vi "SingleServiceRegistered_InvalidResolveRequests_Error.vi"(11 "error in":errorcluster) -> (6 "pass":bool, 8 "result":string, 15 "error out":errorcluster)   [LabVIEW 2020]
uses:
  Runtime/MeasurementLink Discovery Client/RPC Messages/ni_measurementlink_discovery_v1_RegisterServiceRequest.ctl
  Runtime/MeasurementLink Discovery Client/RPC Messages/ni_measurementlink_discovery_v1_ServiceDescriptor.ctl
  Runtime/MeasurementLink Discovery Client/RPC Messages/ni_measurementlink_discovery_v1_ServiceDescriptor_AnnotationsEntry.ctl
  Runtime/MeasurementLink Discovery Client/RPC Messages/ni_measurementlink_discovery_v1_ServiceLocation.ctl
  Runtime/MeasurementLink Discovery Client/RPC Messages/ni_measurementlink_discovery_v1_ResolveServiceRequest.ctl
  Runtime/MeasurementLink Discovery Client/MeasurementLink Discovery Client.lvlib
  Runtime/MeasurementLink Discovery V1/MeasurementLink Discovery V1.lvlib
panel:
  # "Test assumes discovery service has already been started."
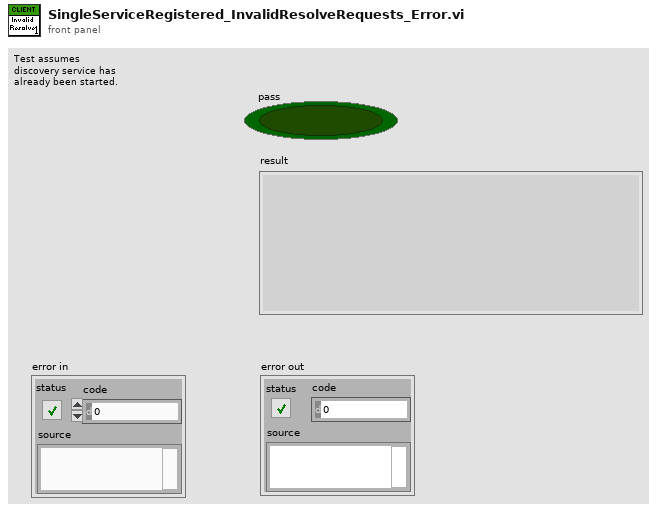
[diagram p1: front panel]
types:
  T1 = typedef "MeasurementLink Discovery Client.lvlib/ni_measurementlink_discovery_v1_ResolveServiceRequest.ctl" = cluster{"provided_interface":string, "service_class":string}
  T2 = typedef "MeasurementLink Discovery Client.lvlib/ni_measurementlink_discovery_v1_RegisterServiceRequest.ctl" = cluster{"service_description":T3, "location":T5}
  T3 = typedef "MeasurementLink Discovery Client.lvlib/ni_measurementlink_discovery_v1_ServiceDescriptor.ctl" = cluster{"display_name":string, "description_url":string, "provided_interfaces":string[], "service_class":string, "annotations":T4[]}
  T4 = typedef "MeasurementLink Discovery Client.lvlib/ni_measurementlink_discovery_v1_ServiceDescriptor_AnnotationsEntry.ctl" = cluster{"key":string, "value":string}
  T5 = typedef "MeasurementLink Discovery Client.lvlib/ni_measurementlink_discovery_v1_ServiceLocation.ctl" = cluster{"location":string, "insecure_port":string, "ssl_authenticated_port":string}
  T6 = typedef "MeasurementLink Discovery Client.lvlib/ni_measurementlink_discovery_v1_RegisterServiceResponse.ctl" = cluster{"registration_id":string}
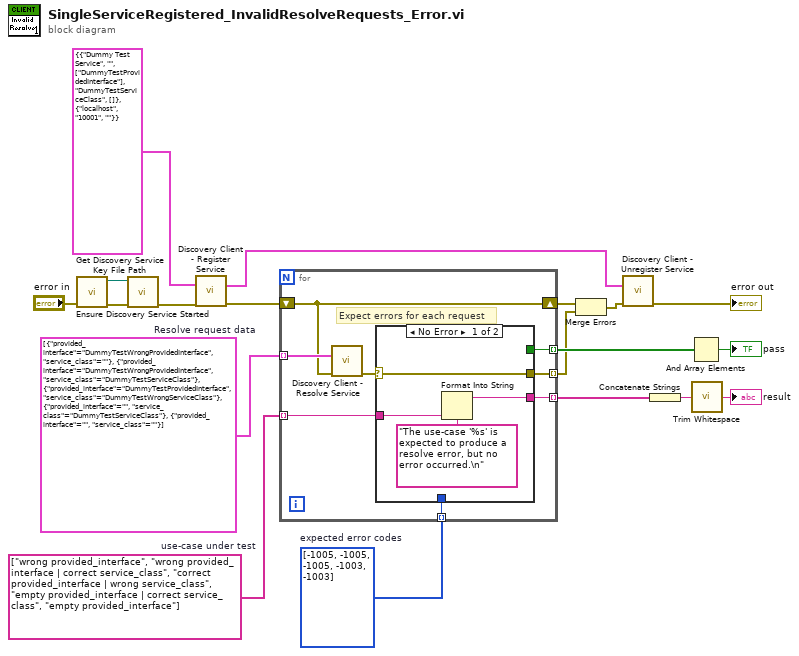
[diagram p0: block diagram]
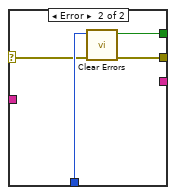
[diagram p2: hidden frame]
diagram:
  w6 = string[] ["wrong provided_interface", "wrong provided_interface | correct service_class", "correct provided_interface | wrong service_class", "empty provided_interface | correct service_class", "empty provided_interface"]  # use-case under test
  w12 = i32[] [-1005, -1005, -1005, -1003, -1003]  # expected error codes
  w15 = T1[] [{"provided_interface"="DummyTestWrongProvidedInterface", "service_class"=""}, {"provided_interface"="DummyTestWrongProvidedInterface", "service_class"="DummyTestServiceClass"}, {"provided_interface"="DummyTestProvidedInterface", "service_class"="DummyTestWrongServiceClass"}, {"provided_interface"="", "service_class"="DummyTestServiceClass"}, {"provided_interface"="", "service_class"=""}]  # Resolve request data
  n1 = call "Get Discovery Service Key File Path.vi"("error in"="error in") -> ("error out"=w4:errorcluster, "key file path"=w3:path)  [unwired: 9 in]
  n2 = call "Ensure Discovery Service Started.vi"("error in"=w4, "path"=w3) -> ("error out"=w2:errorcluster)  [unwired: 8 in, 1 out]
  n3 = call "Discovery Client - Register Service.vi"("Request Data"=T2 {"service_description"={"display_name"="Dummy Test Service", "description_url"="", "provided_interfaces"=["DummyTestProvidedInterface"], "service_class"="DummyTestServiceClass", "annotations"=[]}, "location"={"location"="localhost", "insecure_port"="10001", "ssl_authenticated_port"=""}}, "error in (no error)"=w2) -> ("Response Data"=w19:T6, "error out"=w17:errorcluster)  [unwired: 12 in]
  n4 = for {
    tunnel: w15 -> [w27] mode=indexing
    shift-right: [w26] -> w11
    shift-left: w17 -> [w26]
    tunnel: [w22] -> w13 mode=indexing
    tunnel: w12 -> [w24] mode=indexing
    tunnel: [w23] -> w9 mode=indexing
    tunnel: w6 -> [w21] mode=indexing
    tunnel: [w20] -> w5 mode=indexing
    # "Expect errors for each request"
    n5 = call "Discovery Client - Resolve Service.vi"("Request Data"=w27, "error in (no error)"=w26) -> ("error out"=w25:errorcluster)  [unwired: 12 in, 1 out]
    n6 = case shown="No Error" w25 {
      selector: w25 -> [w31 w32]
      tunnel: [_ w35] -> w22
      tunnel: [w31 w34] -> w23
      tunnel: w24 -> [_ w33]
      tunnel: w21 -> [w29 _]
      tunnel: [w28 _] -> w20
      frame No Error {
        n7 = Format Into String(format string="The use-case '%s' is expected to produce a resolve error, but no error occurred.\n", w29) -> (resulting string=w28:string)  [unwired: 2 in, 1 out]
      }
      frame Error {
        n8 = call <vilib>:"Clear Errors.vi"("error in (no error)"=w32, "specific error code to clear (0: all)"=w33) -> ("error out"=w34:errorcluster, "specific error cleared?"=w35:bool)  [unwired: 4 in]
      }
    }
  }
  n9 = Merge Errors(w11, w9) -> (w10:errorcluster)
  n10 = call "Discovery Client - Unregister Service.vi"("Request Data"=w19, "error in (no error)"=w10) -> ("error out"=→"error out":errorcluster)  [unwired: 12 in, 1 out]
  n11 = Concatenate Strings(w5) -> (w8:string)
  n12 = And Array Elements(Boolean array=w13) -> (logical AND=→"pass":bool)
  n13 = call <vilib>:"Trim Whitespace.vi"("string"=w8) -> ("trimmed string"=→"result":string)  [unwired: 1 in]
